vi "Read Event Data.vi"(8 "error in (no error)":errorcluster, 11 "Receive and Broadcast Event Msg in":refnum<class "Receive and Broadcast Event Msg.lvclass">) -> (0 "error out":errorcluster, 2 "Event Source.lvlib:Event":refnum<class "Event.lvclass">, 3 "Receive and Broadcast Event Msg out":refnum<class "Receive and Broadcast Event Msg.lvclass">)   [LabVIEW 2016, in "Event Source.lvlib" / "Receive and Broadcast Event Msg.lvclass"]
uses:
  Receive and Broadcast Event Msg.lvclass
  Event/Event.lvclass
  Receive and Broadcast Event Msg.lvclass/Receive and Broadcast Event Msg.ctl
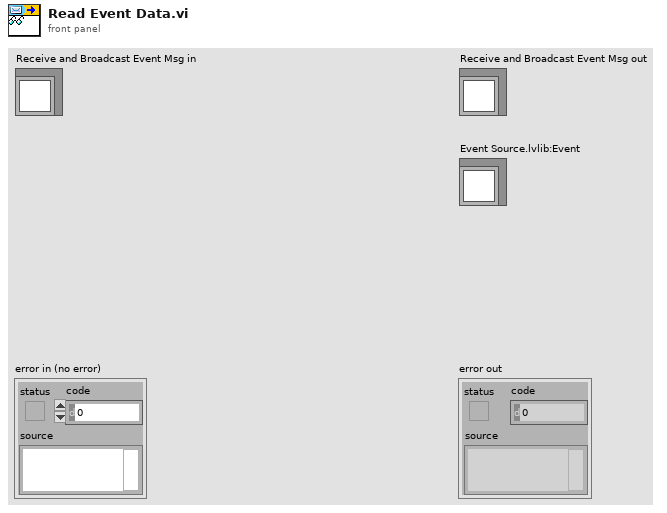
[diagram p1: front panel]
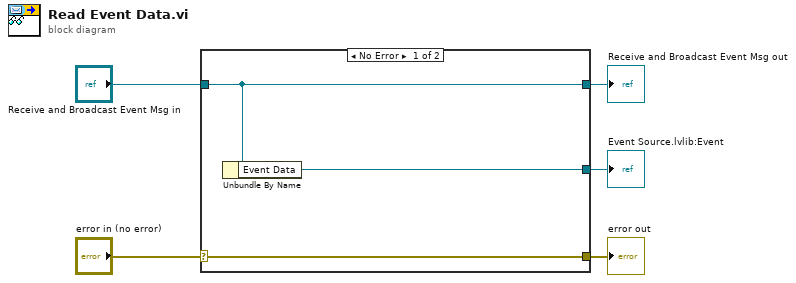
[diagram p0: block diagram]
diagram:
  n1 = case shown="No Error" "error in (no error)" {
    selector: "error in (no error)" -> [w8 w9]
    tunnel: [w8 w9] -> w4
    tunnel: [w7 w10] -> w2
    tunnel: "Receive and Broadcast Event Msg in" -> [w7 w10]
    tunnel: [w6 _] -> w1
    frame No Error {
      n2 = Unbundle By Name(w7) -> ("Event Data"=w6:refnum<class "Event.lvclass">)
    }
    frame Error {
    }
  }
  "error out" <- w4
  "Receive and Broadcast Event Msg out" <- w2
  "Event Source.lvlib:Event" <- w1
